vi "Initialize Test.vi"(6 "Test Index":i32, 8 "error in (no error)":errorcluster, 11 "SV B-M in":refnum<class "SV B-M (Host).lvclass">) -> (0 "error out":errorcluster, 3 "SV B-M out":refnum<class "SV B-M (Host).lvclass">, 5 "Test In Progress":string)   [LabVIEW 2015, in "SV B-M (Host).lvclass"]
doc: "Update the active test index class field and create the info for the test in progress indicator."
uses:
  SV B-M (Host).lvclass
  SV B-M (Host).lvclass/SV B-M (Host).ctl
  Listbox - In Progress.vi
  Listbox - Complete.vi
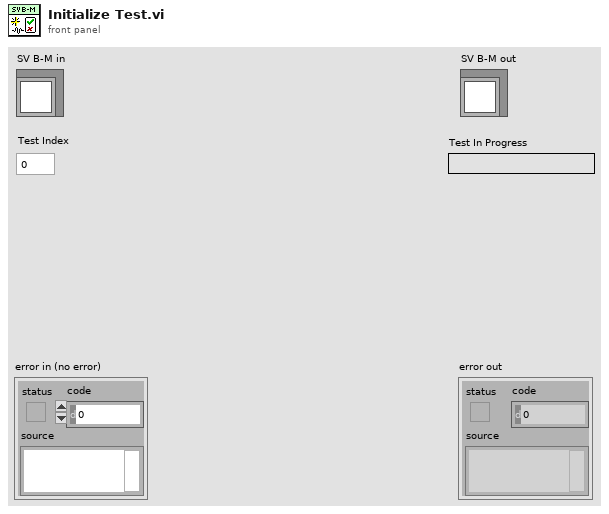
[diagram p1: front panel]
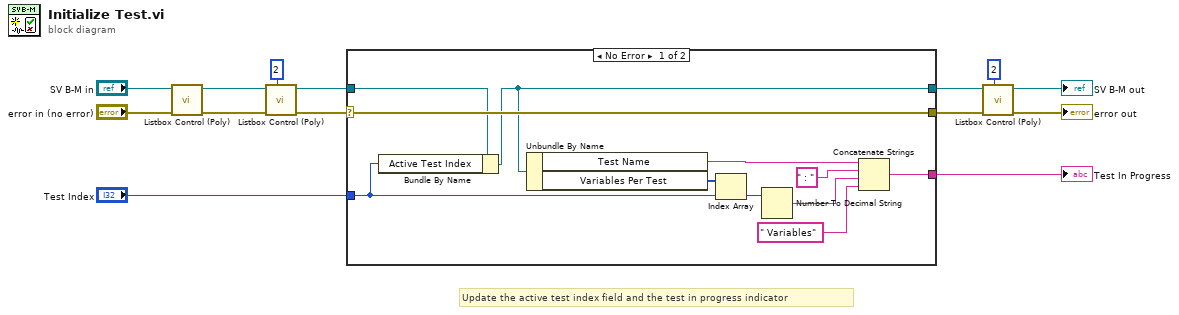
[diagram p0: block diagram]
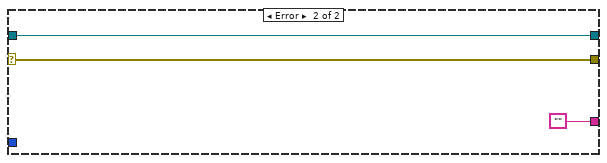
[diagram p2: hidden frame]
diagram:
  # "Update the active test index field and the test in progress indicator"
  n1 = call-poly "Listbox Control (Poly).vi"("error in (no error)"="error in (no error)", "SV B-M In"="SV B-M in") -> ("error out"=w3:errorcluster, "SV B-M Out"=w4:refnum<class "SV B-M (Host).lvclass">)  [unwired: 8 in]
  n2 = call-poly "Listbox Control (Poly).vi"("Row to Update"=2, "error in (no error)"=w3, "SV B-M In"=w4) -> ("error out"=w11:errorcluster, "SV B-M Out"=w13:refnum<class "SV B-M (Host).lvclass">)  [unwired: 7 in]
  n3 = case shown="No Error" w11 {
    selector: w11 -> [w25 w28]
    tunnel: [w25 w28] -> w9
    tunnel: [w23 w27] -> w10
    tunnel: w13 -> [w24 w27]
    tunnel: "Test Index" -> [w22 _]
    tunnel: [w15 ""] -> w14
    frame No Error {
      n4 = Bundle By Name(cluster=w24, "Active Test Index"=w22) -> (w23:refnum<class "SV B-M (Host).lvclass">)
      n5 = Unbundle By Name(w23) -> ("Test Name"=w19:string, "Variables Per Test"=w21:u32[])
      n6 = Index Array(array=w21, index=w22) -> (element=w20:u32)
      n7 = Number To Decimal String(number=w20) -> (decimal integer string=w17:string)  [unwired: 1 in]
      n8 = Concatenate Strings(w19, " : ", w17, " Variables") -> (w15:string)
    }
    frame Error {
    }
  }
  "Test In Progress" <- w14
  n9 = call-poly "Listbox Control (Poly).vi"("Row to Update"=2, "error in (no error)"=w9, "SV B-M In"=w10) -> ("error out"=→"error out":errorcluster, "SV B-M Out"=→"SV B-M out":refnum<class "SV B-M (Host).lvclass">)  [unwired: 7 in]
